vi "Read all.vi"() -> ()   [LabVIEW 2013]
doc: "This example shows how to configure a measurement and take a reading."
uses:
  <vilib>/Utility/file.llb/Read From Spreadsheet File (DBL).vi
  <instrlib>/Keithley 24XX/Public/Data/Read (Single Point).vi
  <vilib>/Utility/file.llb/Write To Spreadsheet File (DBL).vi
  <instrlib>/Keithley 24XX/Keithley 24XX.lvlib
  <vilib>/gmath/NI_Gmath.lvlib
panel:
  in  "文件路径输入":path
  out "幅值-温度":cluster{dbl[], dbl[]}(graph)
  in  "Amp.":dbl[](array[numeric])
  in  "Temp.":dbl[](array[numeric])
  in  "freq.":dbl[](array[numeric])
  out "频率-温度":cluster{dbl[], dbl[]}(graph)
  out "幅值-时间":dbl(graph)
  out "峰频-时间":dbl(graph)
  in  "Network Analyzer\nVISA resource name":refnum<visa-resource-name>
  in  "测量间隔（毫秒）":dbl
  out "温度-时间":dbl(graph)
  out "Temp。":dbl
  in  "定标文件":string(combo)="original.txt"
  in  "Source Mode  (0: Voltage)":u16(ring) items=["Voltage", "Current"]
  in  "Compliance  Level (0.1)":dbl=0.0001
  in  "Output Level (0)":dbl=0.002
  in  "Resistance Auto Range":bool=TRUE
  in  "Current Auto Range":bool=TRUE
  in  "Voltage Auto Range":bool=TRUE
  in  "Resistance Manual Range (1.0)":dbl=1.0
  in  "Current Manual Range (1.0)":dbl=1.0
  in  "Voltage Manual Range (1.0)":dbl=1.0
  out "R":sgl
  out "Curr.":sgl
  out "Vol。":sgl
  in  "Serial Configuration":T1={"Baud Rate"=9600, "Parity"=0, "Data Bits"=8, "Stop Bits"=10, "Flow Control"=0} {"Flow Control" items=["None", "XON/XOFF", "RTS/CTS", "XON/XOFF & RTS/CTS", "DTR/DSR", "XON/XOFF & DTR/DSR"]; "Stop Bits" items=["1.0"=10, "1.5"=15, "2.0"=20]; "Data Bits" items=["7"=7, "8"=8]; "Parity" items=["None", "Odd", "Even", "Mark", "Space"]; "Baud Rate" items=["300"=300, "600"=600, "1200"=1200, "2400"=2400, "4800"=4800, "9600"=9600, "19200"=19200]}
  in  "Keithley 2400\nVISA resource name":refnum<visa-resource-name>
  # "多测量（Keithley 2400 and 5061B） 版本：1.0"
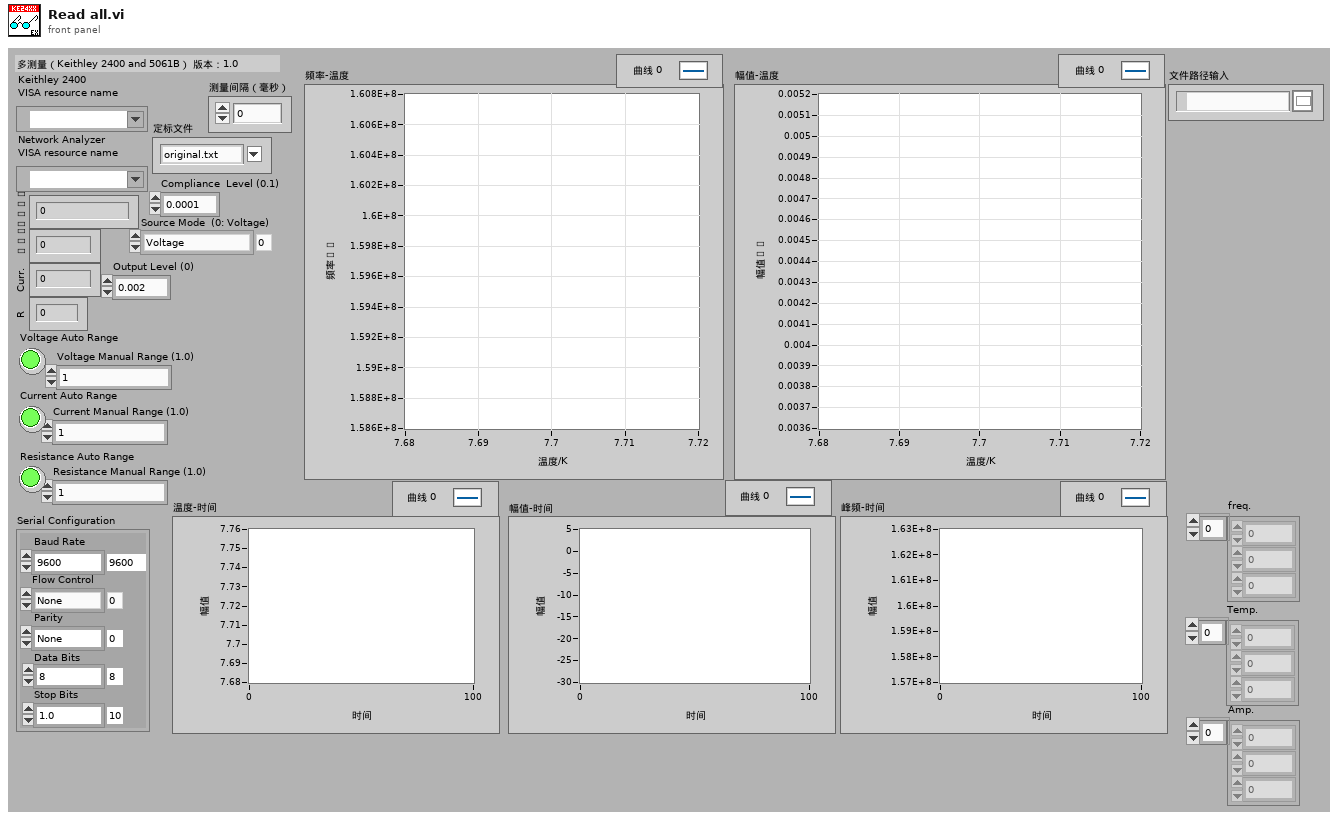
[diagram p1: front panel]
types:
  T1 = cluster{"Baud Rate":u32, "Parity":u16, "Data Bits":u16, "Stop Bits":u16, "Flow Control":u16}
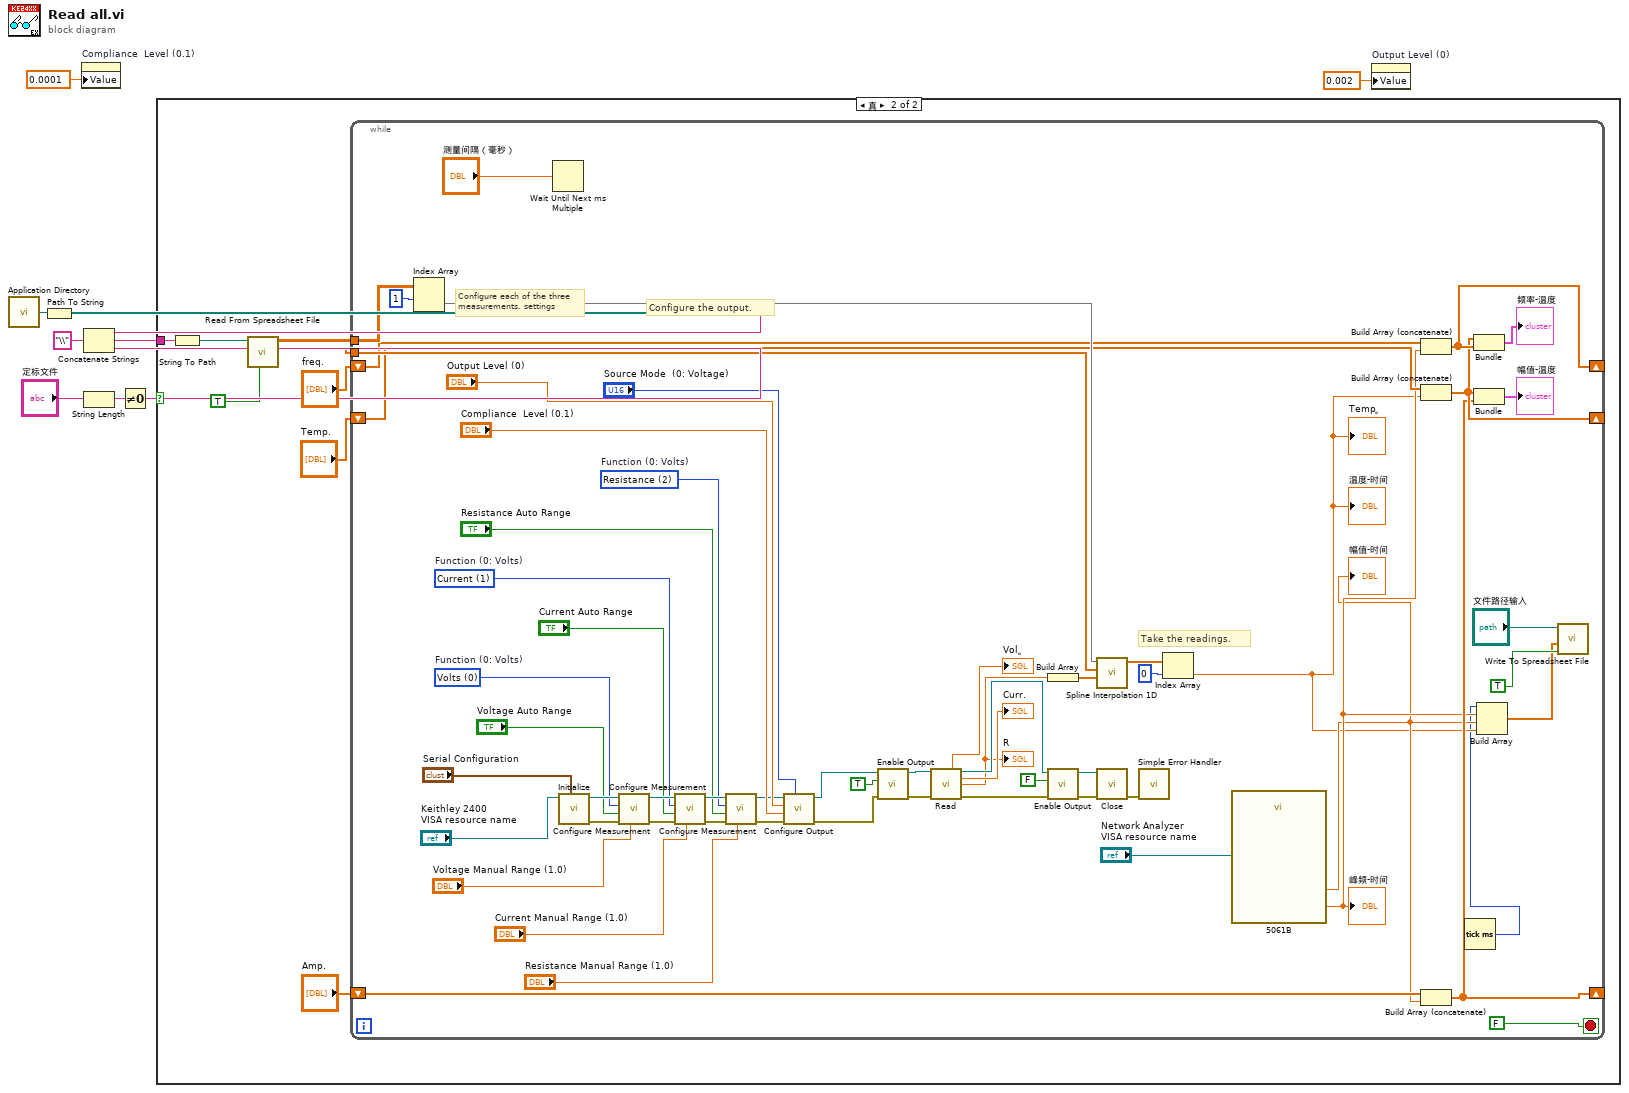
[diagram p0: block diagram]
diagram:
  n1 = call <vilib>:"Application Directory.vi"() -> ("Application Directory"=w9:path)
  n2 = Path To String(path=w9) -> (string=w8:string)
  n3 = property on="Compliance  Level (0.1)" class="DigNum (严格)"("Value"=0.0001) -> ()  [unwired: 2 in, 2 out]
  n4 = Concatenate Strings(w8, "\\", "定标文件") -> (w3:string)
  n5 = String Length(string="定标文件") -> (length=w5:i32)
  n6 = Not Equal To 0?(x=w5) -> (x != 0?=w4:bool)
  n7 = case shown="真" w4 {
    tunnel: w3 -> [_ w13]
    frame False {
    }
    frame True {
      n8 = String To Path(string=w13) -> (path=w17:path)
      n9 = call-poly <vilib>:"Read From Spreadsheet File.vi"("transpose (no:F)"=TRUE, "file path (dialog if empty)"=w17) -> ("first row"=w14:dbl[], "all rows"=w15:dbl[][])  [unwired: 5 in, 3 out]
      n10 = while {
        tunnel: w15 -> [w43]
        tunnel: w14 -> [w42]
        shift-right: [w29] -> _
        shift-left: "freq." -> [w32]
        shift-right: [w27] -> _
        shift-left: "Temp." -> [w31]
        shift-right: [w26] -> _
        shift-left: "Amp." -> [w28]
        stop <- FALSE stop-if-true
        w65 = u16 2 items=["Volts", "Current", "Resistance"]  # Function (0: Volts)
        w66 = u16 1 items=["Volts", "Current", "Resistance"]  # Function (0: Volts)
        w67 = u16 0 items=["Volts", "Current", "Resistance"]  # Function (0: Volts)
        # "Take the readings."
        # "Configure the output."
        # "Configure each of the three measurements. settings"
        n11 = Index Array(array=w43, index (row)=1) -> (element=w41:dbl[])  [unwired: 1 in]
        n12 = Wait Until Next ms Multiple(millisecond multiple="测量间隔（毫秒）") -> ()  [unwired: 1 out]
        n13 = call <instrlib>:"Initialize.vi"("Serial Configuration"="Serial Configuration", "VISA resource name"="Keithley 2400\nVISA resource name") -> ("error out"=w72:errorcluster, "VISA resource name out"=w73:refnum<visa-resource-name>)  [unwired: 8 in]
        n14 = call <instrlib>:"Configure Measurement.vi"("Manual Range (1.0)"="Voltage Manual Range (1.0)", "error in (no error)"=w72, "Enable Auto Range (T:Enable)"="Voltage Auto Range", "Function (0: Volts)"=w67, "VISA resource name"=w73) -> ("error out"=w70:errorcluster, "VISA resource name out"=w71:refnum<visa-resource-name>)  [unwired: 5 in]
        n15 = call <instrlib>:"Configure Measurement.vi"("Manual Range (1.0)"="Current Manual Range (1.0)", "error in (no error)"=w70, "Enable Auto Range (T:Enable)"="Current Auto Range", "Function (0: Volts)"=w66, "VISA resource name"=w71) -> ("error out"=w69:errorcluster, "VISA resource name out"=w68:refnum<visa-resource-name>)  [unwired: 5 in]
        n16 = call <instrlib>:"Configure Measurement.vi"("Manual Range (1.0)"="Resistance Manual Range (1.0)", "error in (no error)"=w69, "Enable Auto Range (T:Enable)"="Resistance Auto Range", "Function (0: Volts)"=w65, "VISA resource name"=w68) -> ("error out"=w46:errorcluster, "VISA resource name out"=w45:refnum<visa-resource-name>)  [unwired: 5 in]
        n17 = call <instrlib>:"Configure Output.vi"("Source Mode  (0: Voltage)"="Source Mode  (0: Voltage)", "error in (no error)"=w46, "Compliance  Level (0.1)"="Compliance  Level (0.1)", "Output Level (0)"="Output Level (0)", "VISA resource name"=w45) -> ("error out"=w48:errorcluster, "VISA resource name out"=w49:refnum<visa-resource-name>)  [unwired: 5 in]
        n18 = call <instrlib>:"Enable Output.vi"("error in (no error)"=w48, "Enable Output (T: Enable)"=TRUE, "VISA resource name"=w49) -> ("error out"=w51:errorcluster, "VISA resource name out"=w50:refnum<visa-resource-name>)  [unwired: 7 in]
        n19 = call-poly <instrlib>:"Read.vi"("VISA resource name"=w50, "error in (no error)"=w51) -> ("Voltage"=→"Vol。":sgl, "VISA resource name out"=w52:refnum<visa-resource-name>, "Current"=→"Curr.":sgl, "Resistance"=w40:sgl, "error out"=w53:errorcluster)  [unwired: 7 in, 2 out]
        "R" <- w40
        n20 = Build Array(w40) -> (w39:sgl[])
        n21 = call <instrlib>:"Enable Output.vi"("error in (no error)"=w53, "Enable Output (T: Enable)"=FALSE, "VISA resource name"=w52) -> ("error out"=w54:errorcluster, "VISA resource name out"=w55:refnum<visa-resource-name>)  [unwired: 7 in]
        n22 = call <vilib>:"Spline Interpolation 1D.vi"("xi"=w39, "X"=w42, "Y"=w41) -> ("yi"=w38:dbl[])  [unwired: 6 in, 2 out]
        n23 = call <instrlib>:"Close.vi"("error in (no error)"=w54, "VISA resource name"=w55) -> ("error out"=w78:errorcluster)  [unwired: 9 in]
        n24 = call <vilib>:"Simple Error Handler.vi"("error in (no error)"=w78) -> ()  [unwired: 4 in, 5 out]
        n25 = Index Array(array=w38, index=0) -> (element=w20:dbl)
        "Temp。" <- w20
        "温度-时间" <- w20
        n26 = call "5061B"("5061B Address"="Network Analyzer\nVISA resource name") -> ("data0"=w21:dbl, "value"=w22:dbl)  [unwired: 23 in, 2 out]
        "峰频-时间" <- w22
        "幅值-时间" <- w21
        n27 = Build Array (concatenate)(w32, w22) -> (w29:dbl[])
        n28 = Build Array (concatenate)(w31, w20) -> (w27:dbl[])
        n29 = Build Array (concatenate)(w28, w21) -> (w26:dbl[])
        n30 = Tick Count (ms)() -> (millisecond timer value=w18:u32)
        n31 = Bundle(w27, w29) -> (→"频率-温度":cluster{dbl[], dbl[]})  [unwired: 1 in]
        n32 = Bundle(w27, w26) -> (→"幅值-温度":cluster{dbl[], dbl[]})  [unwired: 1 in]
        n33 = Build Array(w18, w22, w21, w20) -> (w19:dbl[])
        n34 = call-poly <vilib>:"Write To Spreadsheet File.vi"("append to file? (new file:F)"=TRUE, "1D data"=w19, "file path (dialog if empty)"="文件路径输入") -> ()  [unwired: 5 in, 1 out]
      }
    }
  }
  n35 = property on="Output Level (0)" class="DigNum (严格)"("Value"=0.002) -> ()  [unwired: 2 in, 2 out]
